vi "tm_inputtriggeractive_40.vi"(8 "error in (no error)":errorcluster, 9 "Times":i32=1, 10 "Active":i32(ring)=1 items=["Edge"=1, "Level"=2, "Sync Readout"=3, "Point"=4], 11 "Handle in":u32) -> (0 "error out":errorcluster, 3 "Handle out":u32)   [LabVIEW 2023]
uses:
  tmcamcon.dll
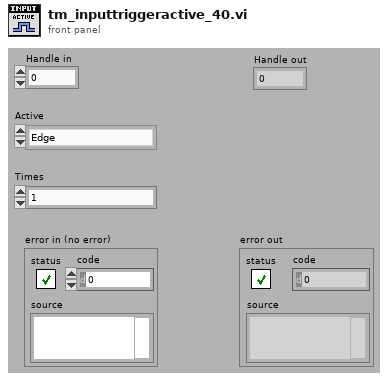
[diagram p1: front panel]
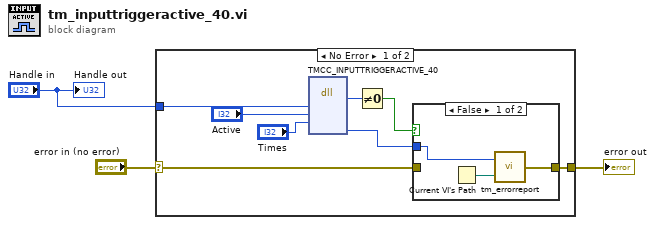
[diagram p0: block diagram]
diagram:
  n1 = case shown="No Error" "error in (no error)" {
    selector: "error in (no error)" -> [w9 w16]
    tunnel: [w6 w16] -> w2
    tunnel: "Handle in" -> [w10 _]
    frame No Error {
      n2 = dll-call lib="tmcamcon.dll" fn="TMCC_INPUTTRIGGERACTIVE_40"("HDCAM"=w10, "active"="Active", "times"="Times") -> ("return type"=w11:u32, "Erval"=w8:i32)  [unwired: 7 in, 2 out]
      n3 = Not Equal To 0?(x=w11) -> (x != 0?=w7:bool)
      n4 = case shown="False" w7 {
        tunnel: w9 -> [_ w15]
        tunnel: [w13 w15] -> w6
        tunnel: w8 -> [w12 _]
        frame False {
          n5 = Current VI's Path() -> (path=w14:path)
          n6 = call "tm_errorreport.vi"("Source"=w14, "Error"=w12) -> ("error out"=w13:errorcluster)
        }
        frame True {
        }
      }
    }
    frame Error {
    }
  }
  "error out" <- w2
  "Handle out" <- "Handle in"
